vi "SIM Propose Step Size.vi"(4 "acceptable err/estimated err":dbl, 5 "error order":i32, 7 "max step size":dbl, 8 "min step size":dbl, 9 "step size":dbl, 10 "proposed step size":dbl, 11 "max step ratio":dbl) -> (2 "proposed step size out":dbl, 3 "proposed max step ratio":dbl)   [LabVIEW 2017]
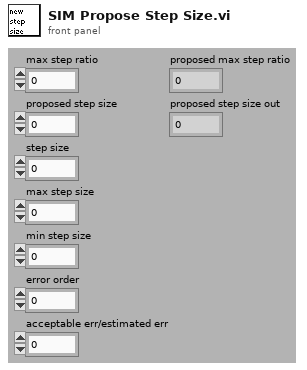
[diagram p1: front panel]
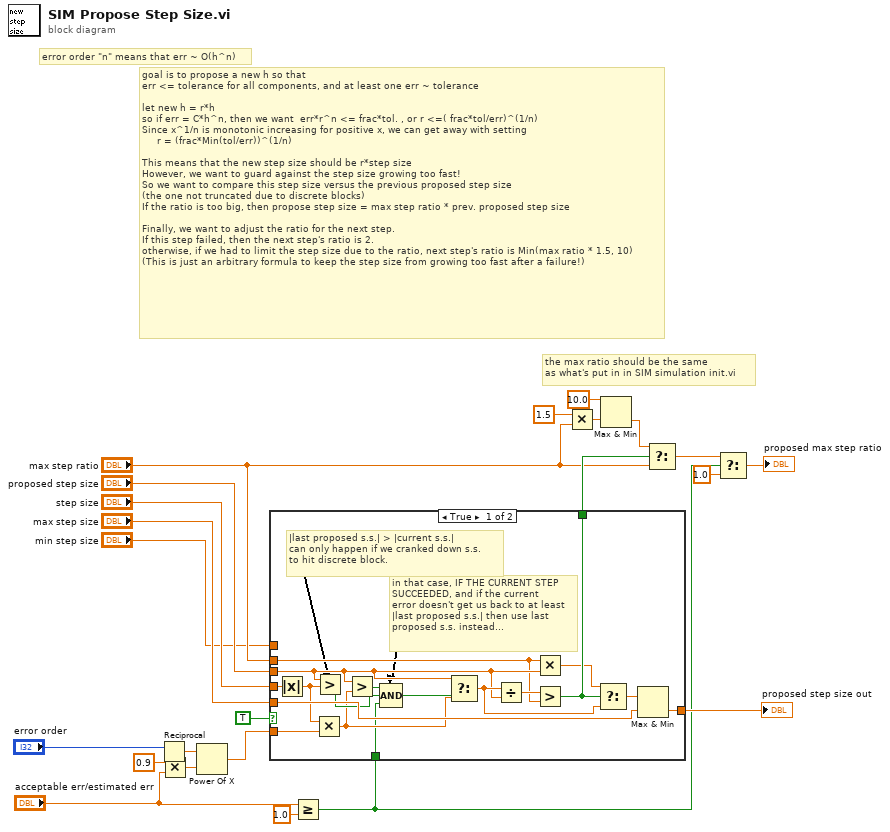
[diagram p0: block diagram]
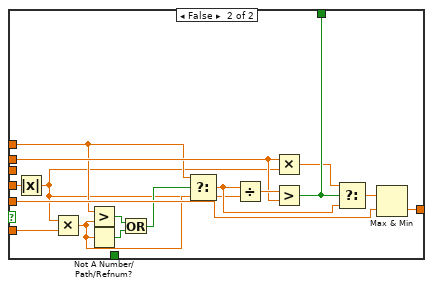
[diagram p2: hidden frame]
diagram:
  # "the max ratio should be the same\nas what's put in in SIM simulation init.vi"
  # "goal is to propose a new h so that \nerr <= tolerance for all components, and at least one err ~ tolerance\n\nlet new h = r*h\nso if err = C*h^n, then we want  err*r^n <= frac*tol. , or r <=( frac*tol/err)^(1/n)\nSince x^1/n is monotonic increasing for positive x, we can get away with setting\n     r = (frac*Min(tol/err))^(1/n)\n\nThis means that the new step size should be r*step size\nHowever, we want to guard against the step size growing too fast!  \nSo we want to compare this step size versus the previous proposed step size \n(the one not truncated due to discrete blocks)\nIf the ratio is too big, then propose step size = max step ratio * prev. proposed step size\n\nFinally, we want to adjust the ratio for the next step.  \nIf this step failed, then the next step's ratio is 2.\notherwise, if we had to limit the step size due to the ratio, next step's ratio is Min(max ratio * 1.5, 10)\n(This is just an arbitrary formula to keep the step size from growing too fast after a failure!)"
  # "error order \"n\" means that err ~ O(h^n)"
  n1 = Reciprocal(x="error order") -> (1/x=w10:dbl)
  n2 = Multiply(x=0.9 ("absolute tolerance"), y="acceptable err/estimated err") -> (x*y=w20:dbl)
  n3 = Power Of X(1:w20, 2:w10) -> (0:w21:dbl)
  n4 = Greater Or Equal?(x="acceptable err/estimated err", y=1.0) -> (x >= y?=w7:bool)
  n5 = case shown="True" TRUE {
    tunnel: w21 -> [w40 w56]
    tunnel: [w39 w55] -> w11
    tunnel: "step size" -> [w36 w52]
    tunnel: [w35 w51] -> w8
    tunnel: "max step size" -> [w33 w49]
    tunnel: w7 -> [w26 _]
    tunnel: "proposed step size" -> [w25 _]
    tunnel: "max step ratio" -> [w24 w47]
    tunnel: "min step size" -> [_ w43]
    frame True {
      # "in that case, IF THE CURRENT STEP\nSUCCEEDED, and if the current\nerror doesn't get us back to at least\n|last proposed s.s.| then use last\nproposed s.s. instead..."
      # "|last proposed s.s.| > |current s.s.|\ncan only happen if we cranked down s.s.\nto hit discrete block."
      n6 = Absolute Value(x=w36) -> (abs(x)=w31:dbl)
      n7 = Multiply(x=w31, y=w40) -> (x*y=w27:dbl)
      n8 = Greater?(x=w25, y=w31) -> (0:w29:bool)
      n9 = Greater?(x=w25, y=w27) -> (0:w30:bool)
      n10 = Compound Arithmetic op=AND(w30, w29, w26) -> (w28:bool)
      n11 = Select(t=w25, s=w28, f=w27) -> (s? t:f=w32:dbl)
      n12 = Divide(x=w32, y=w25) -> (x/y=w37:dbl)
      n13 = Multiply(x=w24, y=w25) -> (x*y=w38:dbl)
      n14 = Greater?(x=w37, y=w24) -> (0:w39:bool)
      n15 = Select(t=w38, s=w39, f=w32) -> (s? t:f=w34:dbl)
      n16 = Max & Min(x=w34, y=w33) -> (min(x,y)=w35:dbl)  [unwired: 1 out]
    }
    frame False {
      n17 = Absolute Value(x=w52) -> (abs(x)=w41:dbl)
      n18 = Multiply(x=w41, y=w56) -> (x*y=w42:dbl)
      n19 = Greater?(x=w43, y=w42) -> (0:w46:bool)
      n20 = Not A Number/Path/Refnum?(number/path/refnum=w42) -> (NaN/Path/Refnum?=w45:bool)
      n21 = Or(x=w46, y=w45) -> (x .or. y?=w44:bool)
      n22 = Select(t=w43, s=w44, f=w42) -> (s? t:f=w48:dbl)
      n23 = Divide(x=w48, y=w41) -> (x/y=w53:dbl)
      n24 = Multiply(x=w47, y=w41) -> (x*y=w54:dbl)
      n25 = Greater?(x=w53, y=w47) -> (0:w55:bool)
      n26 = Select(t=w54, s=w55, f=w48) -> (s? t:f=w50:dbl)
      n27 = Max & Min(x=w50, y=w49) -> (min(x,y)=w51:dbl)  [unwired: 1 out]
    }
  }
  "proposed step size out" <- w8
  n28 = Multiply(x=1.5, y="max step ratio") -> (x*y=w13:dbl)
  n29 = Max & Min(x=10.0, y=w13) -> (min(x,y)=w15:dbl)  [unwired: 1 out]
  n30 = Select(t=w15, s=w11, f="max step ratio") -> (s? t:f=w17:dbl)
  n31 = Select(t=w17, s=w7, f=1.0) -> (s? t:f=→"proposed max step ratio":dbl)
